vi "Test 3 Get Self Distance.vi"(8 "error in (no error)":errorcluster, 11 "Test Case In":refnum<class "Day X Test.lvclass">) -> (0 "error out":errorcluster, 3 "Test Case Out":refnum<class "Day X Test.lvclass">)   [LabVIEW 2020, in "Day X Test.lvclass"]
uses:
  Day X Test.lvclass
  C:/Program Files (x86)/National Instruments/LabVIEW 2020/vi.lib/Astemes/LUnit/Test Case.lvclass
  <vilib>/Astemes/LUnit/Test Case.lvclass/Test Case.ctl
  4993e8ee-a06a-463a-9684-69129f64d5ce.vi
  <vilib>/Astemes/LUnit/Append Pass Result.vi
  <vilib>/Astemes/LUnit/Append Fail Result.vi
  <vilib>/Astemes/LUnit/Describe Comparison.vi
  <vilib>/Astemes/LUnit/Compare Variants.vi
  <vilib>/Astemes/LUnit/Variant to string.vi
  <vilib>/Utility/Data Type/Get Type Information.vi
  <vilib>/Utility/LVClass/Get LV Class Name.vi
  Galaxy/Galaxy.lvclass
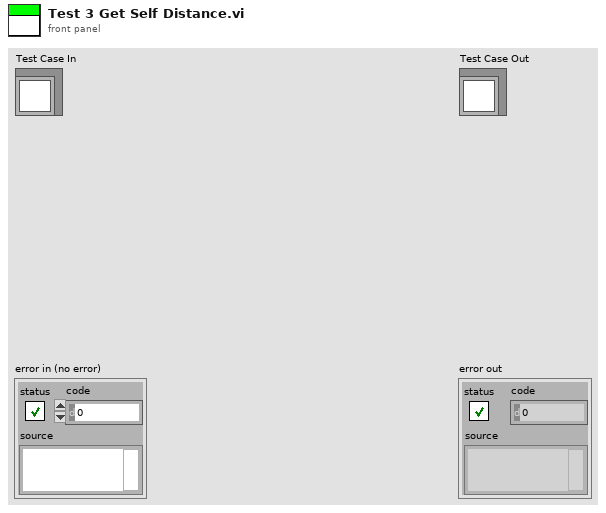
[diagram p1: front panel]
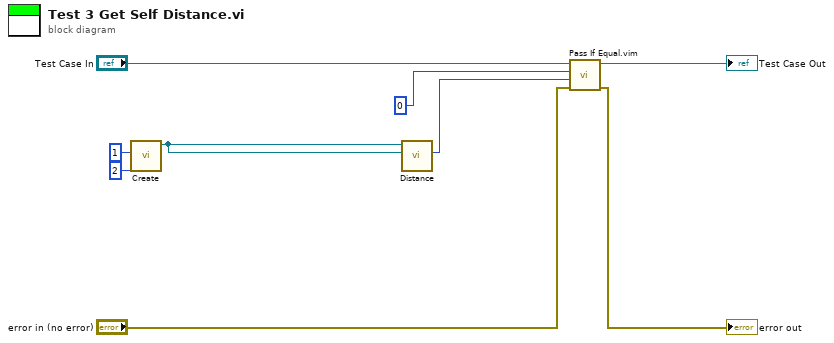
[diagram p0: block diagram]
diagram:
  n1 = call "Create.vi"("Col"=2, "Row"=1) -> ("Galaxy"=w1:refnum<class "Galaxy.lvclass">)  [unwired: 8 in, 1 out]
  n2 = call "Distance.vi"("Galaxy in 2"=w1, "Galaxy in"=w1) -> ("Numeric"=w5:u64)  [unwired: 8 in, 1 out]
  n3 = call "Pass If Equal.vim"("error in (no error)"="error in (no error)", "Actual"=w5, "Expected"=u64 0 ("Numeric"), "LUnit Test Case In"="Test Case In") -> ("error out"=→"error out":errorcluster, "LUnit Test Case Out"=→"Test Case Out":refnum<class "Day X Test.lvclass">)  [unwired: 6 in]
